vi "General_While Loop Stop.vi"(4 "Error In":errorcluster, 5 "Index In":i32=-1, 7 "Array Size In":i32=-1, 8 "Stop 3 In":bool, 9 "Stop 2 In":bool, 10 "Stop 1 In":bool) -> (0 "Stop Out3":bool, 1 "Stop condition":T1=enum."Error", 2 "Stop Out2":bool, 3 "Stop Out1":bool)   [LabVIEW 2014]
uses:
  Controls/Enum/ENUM_General Stop condition.ctl
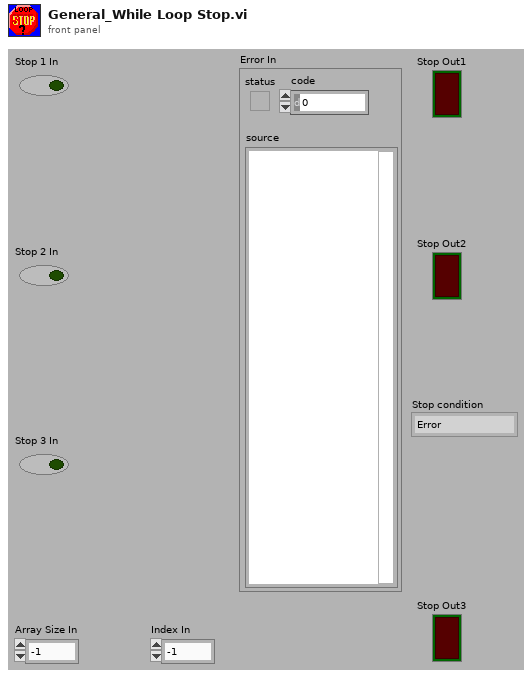
[diagram p1: front panel]
types:
  T1 = typedef "ENUM_General Stop condition.ctl" = enum16{"No Stop", "Error", "Stop 1", "Stop 2", "Stop 3", "Index", "Timeout"}
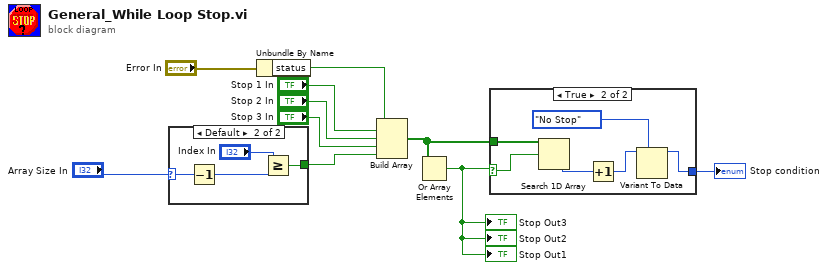
[diagram p0: block diagram]
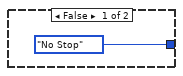
[diagram p2: hidden frame]
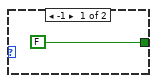
[diagram p3: hidden frame]
diagram:
  n1 = case shown="Default" "Array Size In" {
    selector: "Array Size In" -> [_ w15]
    tunnel: [FALSE w14] -> w8
    frame -1 {
    }
    frame Default {
      n2 = Decrement(x=w15) -> (x-1=w12:i32)
      n3 = Greater Or Equal?(x="Index In", y=w12) -> (x >= y?=w14:bool)
    }
  }
  n4 = Unbundle By Name("Error In") -> ("status"=w4:bool)
  n5 = Build Array(w4, "Stop 1 In", "Stop 2 In", "Stop 3 In", w8) -> (w3:bool[])
  n6 = Or Array Elements(Boolean array=w3) -> (logical OR=w1:bool)
  "Stop Out1" <- w1
  "Stop Out2" <- w1
  "Stop Out3" <- w1
  n7 = case shown="True" w1 {
    selector: w1 -> [_ w21]
    tunnel: w3 -> [_ w22]
    tunnel: [ENUM_General_Stop_condition."No Stop" ("Stop condition") w17] -> w2
    frame False {
    }
    frame True {
      n8 = Search 1D Array(1D array=w22, element=w21) -> (index of element=w20:i32)  [unwired: 1 in]
      n9 = Increment(x=w20) -> (x+1=w19:i32)
      n10 = Variant To Data(type=ENUM_General_Stop_condition."No Stop" ("Stop condition"), Variant=w19) -> (data=w17:T1)  [unwired: 1 in, 1 out]
    }
  }
  "Stop condition" <- w2
